vi "Magnet-RP alignment.vi"() -> ()   [LabVIEW 2016]
uses:
  <vilib>/Waveform/WDTOps.llb/WDT Get Final Time Value DBL.vi
panel:
  out "attributes":variant
  out "Actual start \ntime of Pitaya":timestamp
  in  "delay IV ramps \nafter trigger (points)":i32
  in  "pre IV ramp points":i32
  out "Waveform Graph":waveform(dbl)[](graph)
  out "tf 2":timestamp
  out "dt 2":dbl
  out "t0 2":timestamp
  out "Y 2":dbl[](array[numeric])
  in  "Channel name 2":string="CH0"
  in  "File Path 2":path
  out "tf":timestamp
  out "dt":dbl
  out "t0":timestamp
  out "Y":dbl[](array[numeric])
  in  "Channel name":string="CH0"
  in  "File Path":path
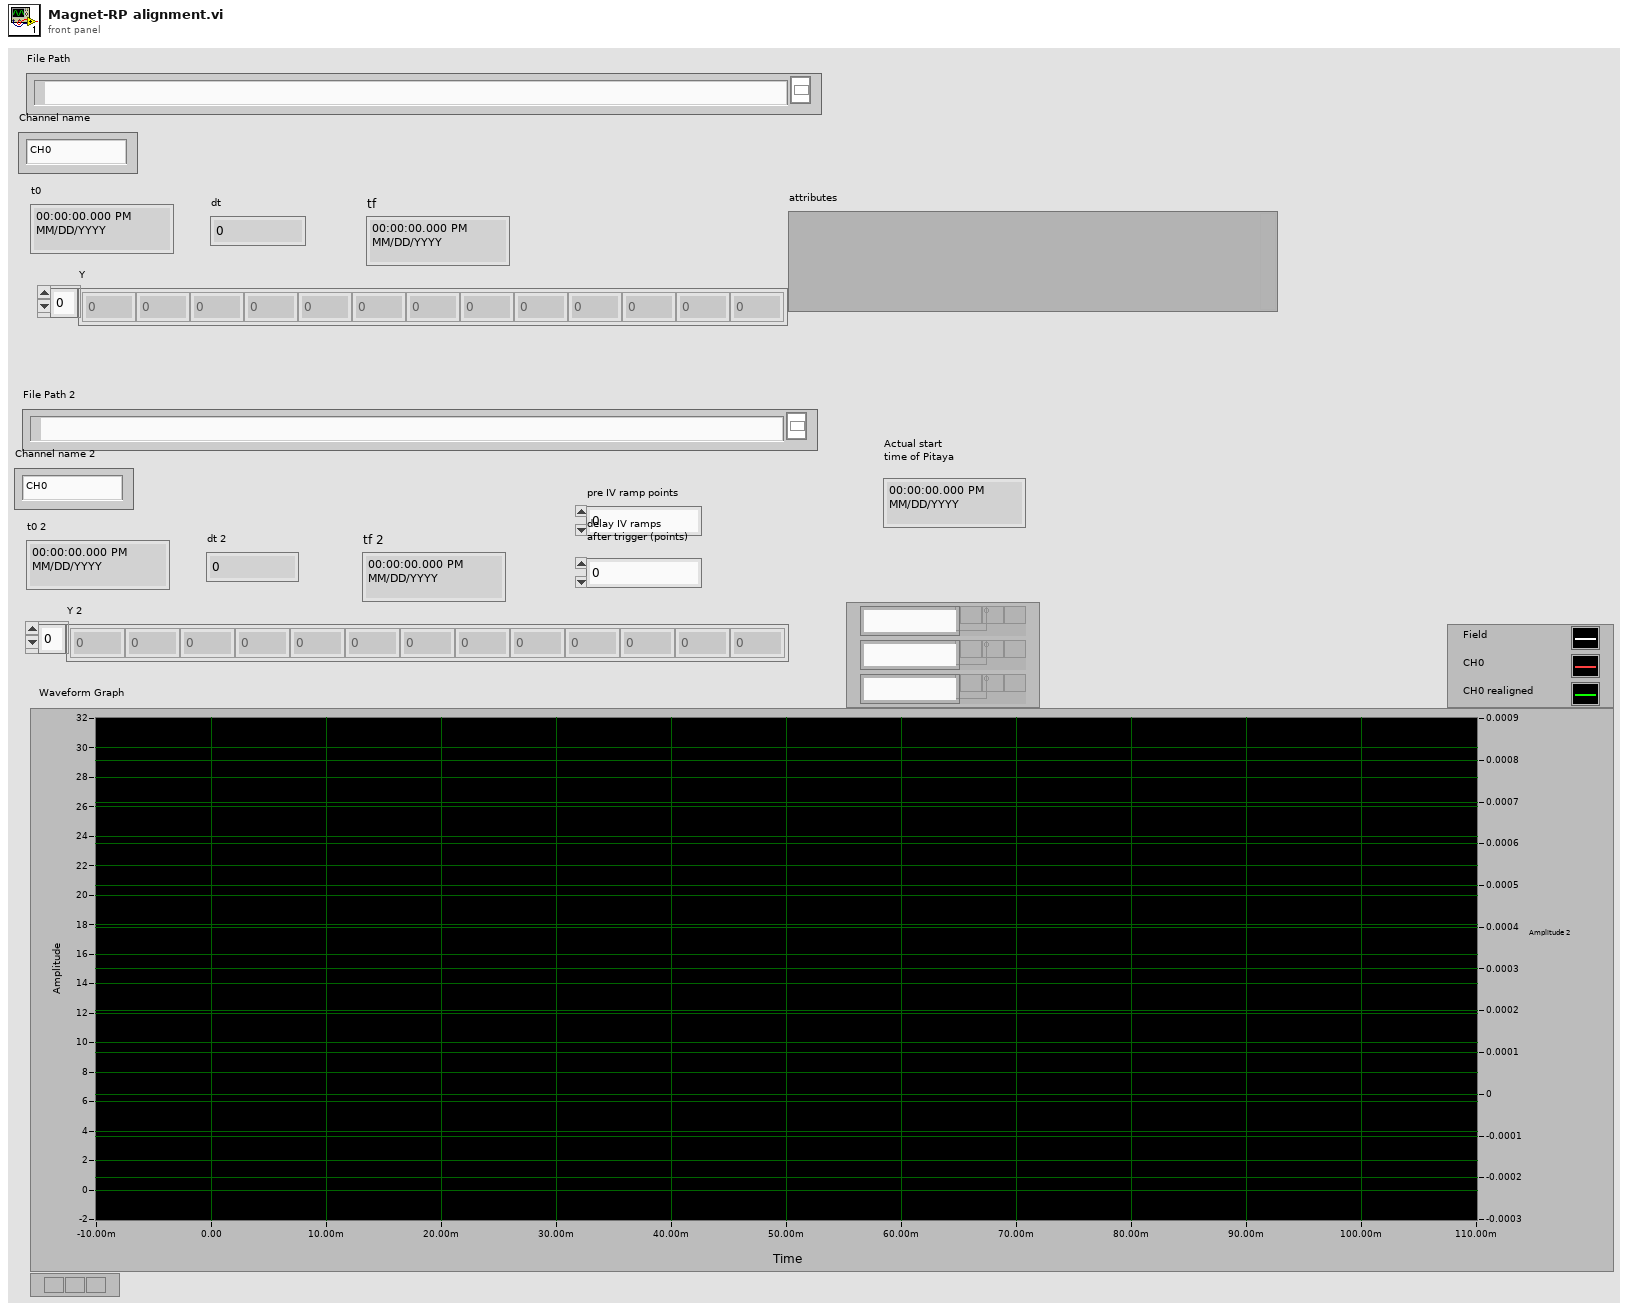
[diagram p1: front panel]
types:
  T1 = enum16{"open", "open or create", "create or replace", "create", "open (read-only)"}
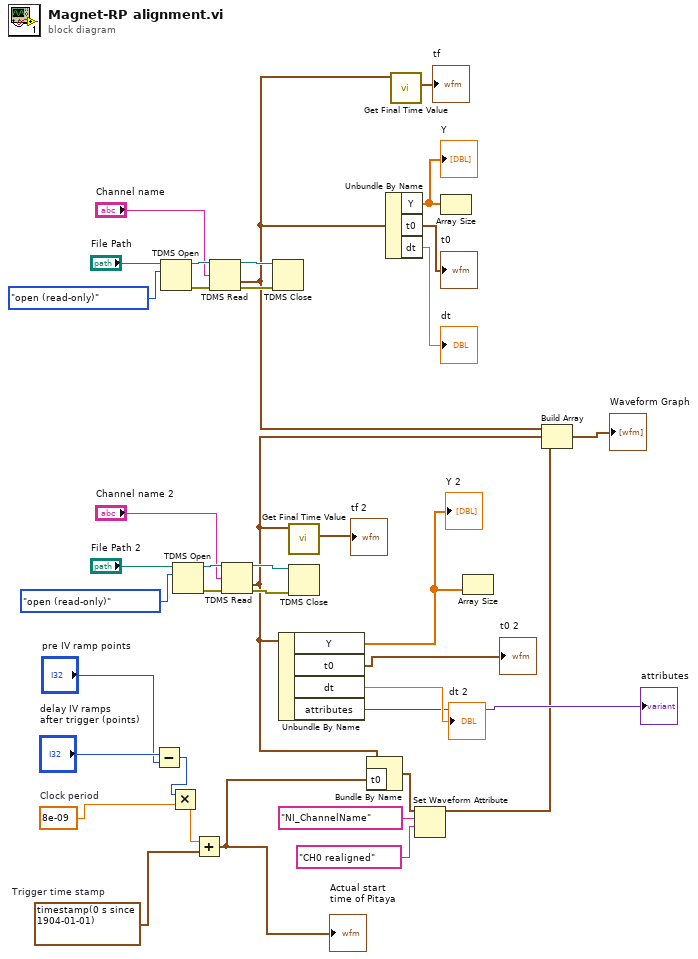
[diagram p0: block diagram]
diagram:
  w9 = timestamp(0.0007999963039997185 s since 1904-01-01)  # Trigger time stamp
  w10 = 8e-09  # Clock period
  n1 = Subtract(x="delay IV ramps \nafter trigger (points)", y="pre IV ramp points") -> (x-y=w11:i32)
  n2 = TDMS Open(10:T1."open (read-only)" ("operation (0:open)"), 11:"File Path") -> (0:w35:errorcluster, 3:w37:refnum<k34>)  [unwired: 5 in]
  n3 = Multiply(x=w11, y=w10) -> (x*y=w8:dbl)
  n4 = TDMS Open(10:T1."open (read-only)" ("operation (0:open)"), 11:"File Path 2") -> (0:w24:errorcluster, 3:w26:refnum<k34>)  [unwired: 5 in]
  n5 = Add(x=w8, y=w9) -> (x+y=w6:timestamp)
  "Actual start \ntime of Pitaya" <- w6
  n6 = TDMS Read(0:w37, 7:"Channel name", 11:w35) -> (4:w36:refnum<k34>, 10:w15:waveform(dbl), 15:w34:errorcluster)  [unwired: 5 in, 3 out]
  n7 = TDMS Read(0:w26, 7:"Channel name 2", 11:w24) -> (4:w25:refnum<k34>, 10:w7:waveform(dbl), 15:w23:errorcluster)  [unwired: 5 in, 3 out]
  n8 = TDMS Close(8:w34, 11:w36) -> ()  [unwired: 2 out]
  n9 = Unbundle By Name(w7) -> ("Y"=w16:dbl[], "t0"=→"t0 2":timestamp, "dt"=→"dt 2":dbl, "attributes"=→"attributes":variant)
  "Y 2" <- w16
  n10 = call-poly <vilib>:"Get Final Time Value.vi"("waveform in"=w7) -> ("tf"=→"tf 2":timestamp)  [unwired: 8 in, 2 out]
  n11 = TDMS Close(8:w23, 11:w25) -> ()  [unwired: 2 out]
  n12 = Bundle By Name(cluster=w7, "t0"=w6) -> (w4:waveform(dbl))
  n13 = Unbundle By Name(w15) -> ("Y"=w28:dbl[], "t0"=→"t0":timestamp, "dt"=→"dt":dbl)
  "Y" <- w28
  n14 = call-poly <vilib>:"Get Final Time Value.vi"("waveform in"=w15) -> ("tf"=→"tf":timestamp)  [unwired: 8 in, 2 out]
  n15 = Set Waveform Attribute(5:"CH0 realigned" ("name"), 6:"NI_ChannelName" ("name"), 7:w4) -> (3:w3:waveform(dbl))  [unwired: 1 in, 2 out]
  n16 = Array Size(array=w28) -> ()  [unwired: 1 out]
  n17 = Array Size(array=w16) -> ()  [unwired: 1 out]
  n18 = Build Array(w15, w7, w3) -> (→"Waveform Graph":waveform(dbl)[])
